vi "GT Pvt Status.vi"(6 "count":i16, 7 "pTime":dbl, 8 "error in (no error)":errorcluster caption="错误输入（无错误）", 9 "pTableId":i16, 10 "profile":i16, 11 "cardNum":i16) -> (0 "error out":errorcluster caption="错误输出", 1 "pTableId out":i16, 3 "function return":i16, 5 "pTime out":dbl)   [LabVIEW 2020, in "gts.lvlib"]
doc: "GT_API GT_PvtStatus(short cardNum,short profile,short *pTableId,double *pTime,short count=1);"
uses:
  gts.lvlib
  dll/32bit/multi_card/gts.dll
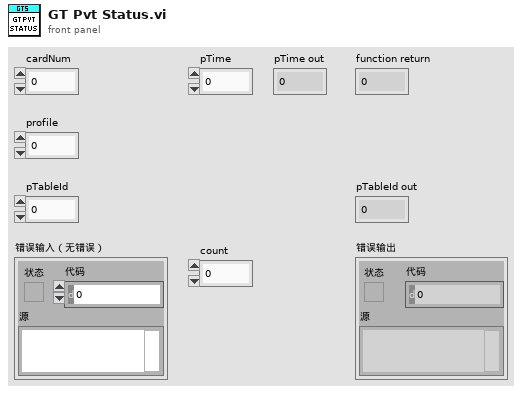
[diagram p1: front panel]
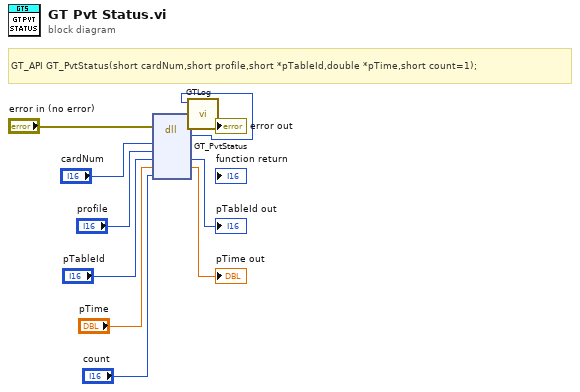
[diagram p0: block diagram]
diagram:
  # "GT_API GT_PvtStatus(short cardNum,short profile,short *pTableId,double *pTime,short count=1);"
  n1 = dll-call lib="C:/1228/dll/32bit/multi_card/gts.dll" fn="GT_PvtStatus"(error in="error in (no error)", "cardNum"="cardNum", "profile"="profile", "pTableId"="pTableId", "pTime"="pTime", "count"="count") -> (error out=w3:errorcluster, w1:i16, "pTableId"=→"pTableId out":i16, "pTime"=→"pTime out":dbl)  [unwired: 5 in, 1 out]
  n2 = call "GTLog.vi"("error in (no error)"=w3, "Numeric"=w1) -> ("error out"=→"error out":errorcluster)  [unwired: 9 in]
